vi "Rename.vi"() -> ()   [LabVIEW 2019]
panel:
  out "element":string
  out "List of Documents":string[][](array[string])
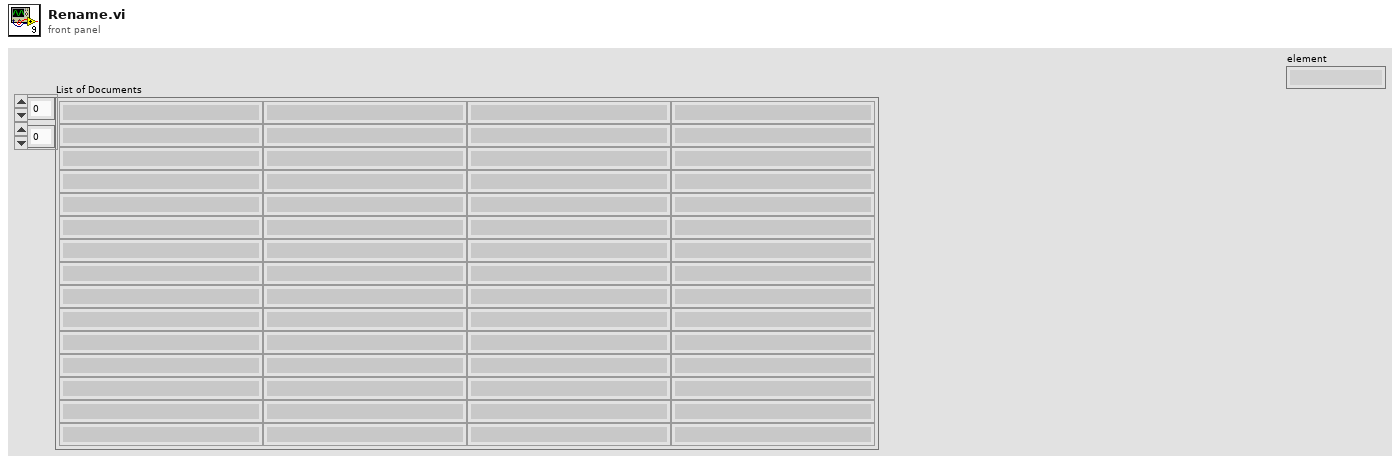
[diagram p1: front panel]
types:
  T1 = cluster{"Date":string, "On-Nonce":string, "ctype":string, "path":string, "method":string, "Authorization":string, "Accept":string, "User-Agent":string, "Content-Type":string, "secret_key":string, "access_key":string, "stack":string, "payload":string, "headers":string[], "eid":string, "wid":string, "did":string, "name":string}
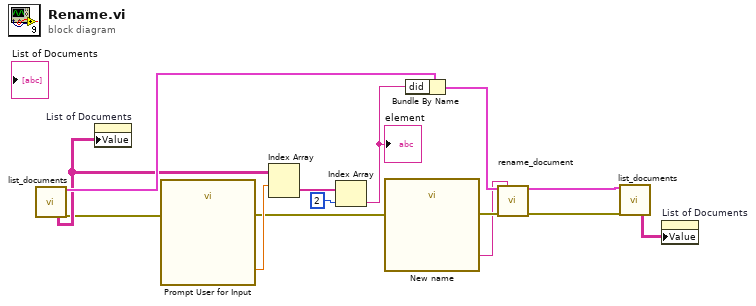
[diagram p0: block diagram]
diagram:
  n1 = call <userlib>:"list_documents.vi"() -> ("Document list"=w7:string[][], "Device Out"=w10:T1, "error out"=w1:errorcluster)  [unwired: 16 in, 1 out]
  n2 = property on="List of Documents" class="Arr (strict)"("Value"=w7) -> ()  [unwired: 2 in, 2 out]
  n3 = call "Prompt User for Input"("error in (no error)"=w1) -> ("SN"=w5:dbl, "error out"=w4:errorcluster)  [unwired: 16 in, 1 out]
  n4 = Index Array(array=w7, index (row)=w5) -> (element=w14:string[])  [unwired: 1 in]
  n5 = Index Array(array=w14, index=2) -> (element=w9:string)
  "element" <- w9
  n6 = call "New name"("error in (no error)"=w4) -> ("New name"=w2:string, "error out"=w3:errorcluster)  [unwired: 16 in, 1 out]
  n7 = Bundle By Name(cluster=w10, "did"=w9) -> (w8:T1)
  n8 = call <userlib>:"rename_document.vi"("Device In"=w8, "Name"=w2, "error in"=w3) -> ("Device Out"=w12:T1, "error out"=w11:errorcluster)  [unwired: 10 in, 1 out]
  n9 = call <userlib>:"list_documents.vi"("Device  In"=w12, "error in"=w11) -> ("Document list"=w6:string[][])  [unwired: 14 in, 3 out]
  n10 = property on="List of Documents" class="Arr (strict)"("Value"=w6) -> ()  [unwired: 2 in, 2 out]
